vi "Climb Teleop Handler.vi"   [LabVIEW 2023]
uses:
  fd08f4e7-806c-4d6c-8ad4-ee12c04251c0.vi
  <vilib>/Rock Robotics/WPI/Utilities/WPI_GetSetVariantRefNum.vi
  Framework/Robot Global Data.vi
types:
  T1 = typedef "WPI_JoystickDevRef.ctl" = cluster{"Device":T2}
  T2 = typedef "WPI_JoystickDeviceEnum.ctl" = enum16{"USB 0", "USB 1", "USB 2", "USB 3", "USB 4", "USB 5"}
  T3 = typedef "Climb Operations.ctl" = enum16{"Reserve", "Read Current", "Idle", "Retract", "Deploy"}
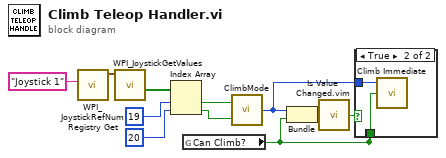
[diagram p0: block diagram]
diagram:
  n1 = call <vilib>:"WPI_JoystickRefNum Registry Get.vi"("refnum name"="Joystick 1") -> ("JoystickDevRef"=w9:T1)  [unwired: 1 in, 9 out]
  n2 = call <vilib>:"WPI_JoystickGetValues.vi"("JoystickDevRef"=w9) -> ("Buttons"=w8:bool[])  [unwired: 6 in, 4 out]
  n3 = Index Array(array=w8, index #1=19 ("index"), index #2=20 ("index")) -> (element #1=w5:bool, element #2=w4:bool)
  n4 = global read "Robot Global Data.vi" "Can Climb?"() -> (w1:bool)
  n5 = call "ClimbMode.vi"("Retract"=w4, "Deploy"=w5) -> ("Climb Mode"=w2:T3)
  n6 = Bundle("Climb Mode"=w2, "Can Climb?"=w1) -> (w3:cluster{"Climb Mode":T3, "Can Climb?":bool})  [unwired: 1 in]
  n7 = call "Is Value Changed.vim"("value"=w3) -> ("changed or first call?"=w11:bool)
  n8 = case shown="True" w11 {
    tunnel: w2 -> [_ w13]
    tunnel: w1 -> [_ _]
    tunnel: w1 -> [_ w12]
    frame False {
    }
    frame True {
      n9 = call "Climb Immediate.vi"("Can Climb?"=w12, "Climb modes"=w13) -> ()  [unwired: 2 in, 1 out]
    }
  }
